vi "Goodbye.vi"(9 "Goodbye Request":T1={"Error URI"="wamp.close.shut_down", "Message"="client disconnect"}, 10 "error in (no error)":errorcluster, 11 "WAMP Client in":refnum<class "WAMP Client.lvclass">) -> (2 "error out":errorcluster, 3 "WAMP Client out":refnum<class "WAMP Client.lvclass">)   [LabVIEW 2020, in "WAMP Client.lvclass"]
uses:
  <userlib>/lvwamp/WAMP Client/WAMP Client.lvclass
  <userlib>/lvwamp/WAMP Client/TypeDef/GOODBYE Request Data.ctl
  <userlib>/lvwamp/WAMP Client/WAMP Client.lvclass/WAMP Client.ctl
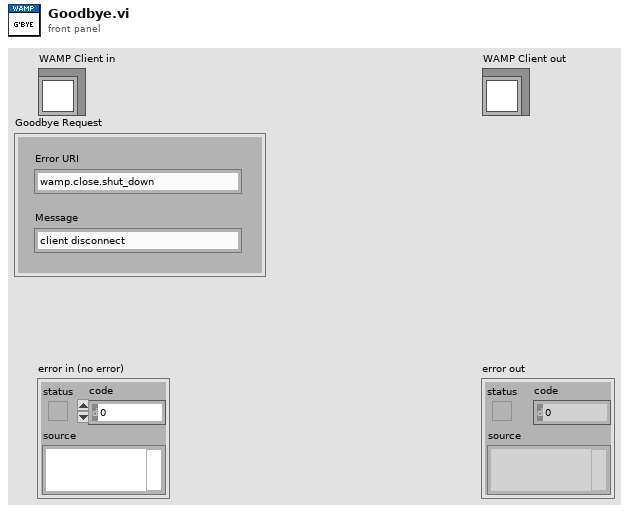
[diagram p1: front panel]
types:
  T1 = typedef "WAMP Client.lvclass/GOODBYE Request Data.ctl" = cluster{"Error URI":string, "Message":string}
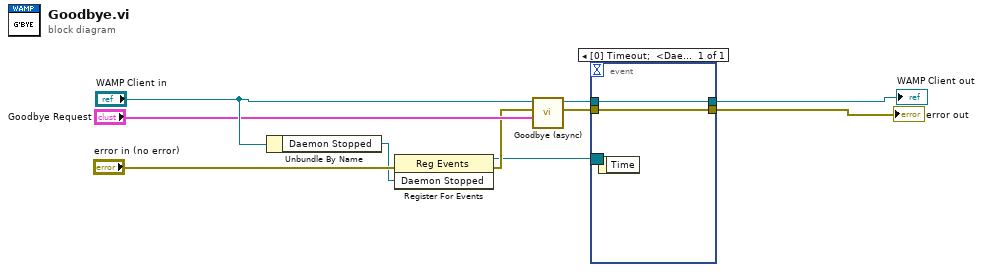
[diagram p0: block diagram]
diagram:
  n1 = Unbundle By Name("WAMP Client in") -> ("Daemon Stopped"=w5:refnum<user-event>)
  n2 = register-events(error in="error in (no error)", w5) -> (reference out=w3:refnum<event-registration>, error out=w4:errorcluster)  [unwired: 1 in]
  n3 = call-dynamic "Goodbye (async).vi"("Goodbye Request"="Goodbye Request", "error in (no error)"=w4, "WAMP Client in"="WAMP Client in") -> ("error out"=w1:errorcluster, "WAMP Client out"=w2:refnum<class "WAMP Client.lvclass">)  [unwired: 7 in]
  n4 = event shown="[0] Timeout;  <Daemon Stopped>: User Event" {
    selector: w3 -> [_]
    dyn-events: _ -> [_]
    timeout: _ -> [_]
    tunnel: w2 -> [w12]
    tunnel: [w12] -> w7
    tunnel: w1 -> [w11]
    tunnel: [w11] -> w9
    event Timeout; User Event {
      n5 = event-data() -> ()  [unwired: 1 in, 1 out]
    }
  }
  "error out" <- w9
  "WAMP Client out" <- w7
